vi "Get Data.vi"(8 "error in (no error)":errorcluster, 11 "Meter Measurement in":refnum<class "Meter Measurement.lvclass">) -> (0 "error out":errorcluster, 3 "Meter Measurement out":refnum<class "Meter Measurement.lvclass">)   [LabVIEW 2015, in "Meter Measurement.lvclass"]
uses:
  Meter Measurement.lvclass
  Meter Measurement.lvclass/Meter Measurement.ctl
  <vilib>/ActorFramework/Message Enqueuer/Message Enqueuer.lvclass/Message Enqueuer.ctl
  <vilib>/ActorFramework/Message Enqueuer/Enqueue.vi
  <vilib>/ActorFramework/Message Priority Queue/Priority Enqueue.vi
  <vilib>/ActorFramework/Message Enqueuer/Message Enqueuer.lvclass
  Mag Lab Hardware Messages/Measure Msg/Measure Msg.lvclass
  Mag Lab Measurement/Mag Lab Measurement.lvclass
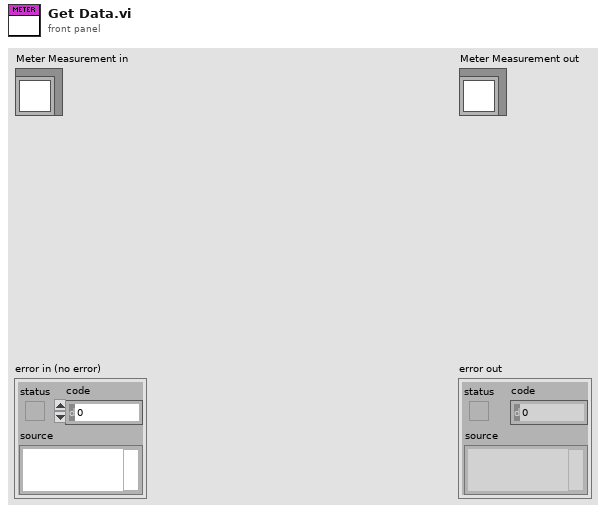
[diagram p1: front panel]
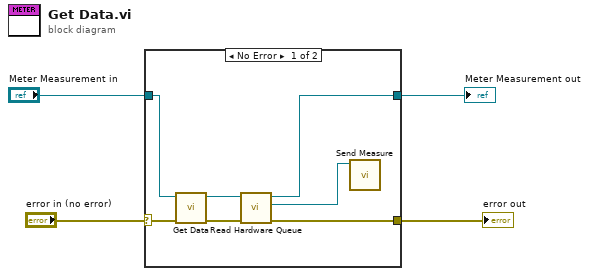
[diagram p0: block diagram]
diagram:
  n1 = case shown="No Error" "error in (no error)" {
    selector: "error in (no error)" -> [w9 w12]
    tunnel: [w6 w12] -> w4
    tunnel: [w8 w13] -> w3
    tunnel: "Meter Measurement in" -> [w10 w13]
    frame No Error {
      n2 = call-parent "Get Data.vi"("error in (no error)"=w9, "Mag Lab Measurement in"=w10) -> ("error out"=w7:errorcluster, "Mag Lab Measurement out"=w11:refnum<class "Meter Measurement.lvclass">)  [unwired: 8 in]
      n3 = call "Read Hardware Queue.vi"("error in (no error)"=w7, "Meter Measurement in"=w11) -> ("error out"=w6:errorcluster, "Actor Framework:Message Enqueuer"=w5:refnum<class "Message Enqueuer.lvclass">, "Meter Measurement out"=w8:refnum<class "Meter Measurement.lvclass">)  [unwired: 7 in]
      n4 = call "Send Measure.vi"("Message Enqueuer"=w5) -> ()  [unwired: 9 in, 2 out]
    }
    frame Error {
    }
  }
  "error out" <- w4
  "Meter Measurement out" <- w3
